vi "Q14070-Z030装调整机构.vi"() -> ()   [LabVIEW 2013]
panel:
  out "error out 4":errorcluster
  out "人工判断不合格状态":bool
  out "涂脂报警状态":string
  out "涂脂报警工步号":dbl
  out "error out 3":errorcluster
  out "型号数量":i32=10
  out "KSJJ":string
  out "FGCS":string
  out "03RFID":string
  out "RFID读取完成":bool
  out "RFID读取触发":bool
  out "芯片ID":string
  out "产品ID":string
  in  "锁紧螺母批次号":string
  in  "调整螺塞批次号":string
  in  "弹簧批次号":string
  in  "O型圈批次号":string
  in  "支撑座批次号":string
  in  "复位按钮":bool
  in  "停止":bool
  in  "联线按钮":bool
  out "通讯状态":bool
  in  "选项卡控件 2":enum32{"自动", "手动", "参数查询"}(tab)
  in  "人工判断\n不合格":bool
  out "本序已做":bool
  out "本序合格":bool
  out "上序不合格":bool
  out "上序合格":bool
  out "取料操作状态":string
  out "取料工步号":dbl
  out "涂脂操作状态":string
  out "涂脂工步号":dbl
  out "流水线操作状态":string
  in  "流水线工步号":dbl
  out "报警提示":string
  out "报警工步号":dbl
  out "I上工位在位":bool
  out "I本工位在位":bool
  out "I下工位在位":bool
  out "I旋转气缸原位  2":bool
  out "I顶升气缸下位 2":bool
  out "I顶升气缸上位  2":bool
  out "I旋转气缸进位 2":bool
  out "I胶瓶在位":bool
  out "I辅具在位":bool
  out "I横孔涂脂在位":bool
  in  "M支撑座手动涂脂有效":bool
  in  "M图像识别涂脂开":bool
  in  "M图像识别触发":bool
  in  "M本工位放行":bool
  in  "M流水线旋转气缸原位":bool
  in  "M上工位放行":bool
  in  "M流水线顶升气缸下降":bool
  in  "M流水线旋转气缸旋转":bool
  in  "M横孔涂脂开":bool
  in  "M流水线顶升气缸顶升":bool
  out "下工位在位":bool
  out "上工位在位":bool
  out "本工位在位":bool
  out "旋转气缸进位":bool
  out "顶升气缸上位":bool
  out "顶升气缸下位":bool
  out "旋转气缸原位":bool
  in  "操作步骤":T1
  in  "参数修改":bool
  in  "参数查询":bool
  in  "参数列表":string[][](table)
  out "员工ID":string
  out "员工姓名":string
  in  "型号选择":u16(ring)=1 items=["J706", "J709", "J728", "J728A", "J728B", "J506X"]
  in  "参数加载":bool
  out "Q场景切换启动2":bool
  out "Q场景切换启动1":bool
  out "备用取料":i16=4
  out "error out 2":errorcluster
  out "ADODB._Connection Out":refnum<k7>
  out "error out":errorcluster
  out "Q场景切换 4":bool
  out "Q场景切换 3":bool
  out "Q场景切换 2":bool
  out "Q场景切换":bool
  out "场景切换选择":i16=4
  out "横孔涂脂设定次数":i16=4
  out "齿条支撑座涂脂设定次数":i16=4
  in  "M备用取料":bool
  out "产品选型":dbl
  # "芜湖机械转向器装配线"
  # "Z030 装调整机构"
  # "Q14070机械转向器装配线"
  # "湖北唯思凌科装备制造有限公司 设计开发 (C)2015"
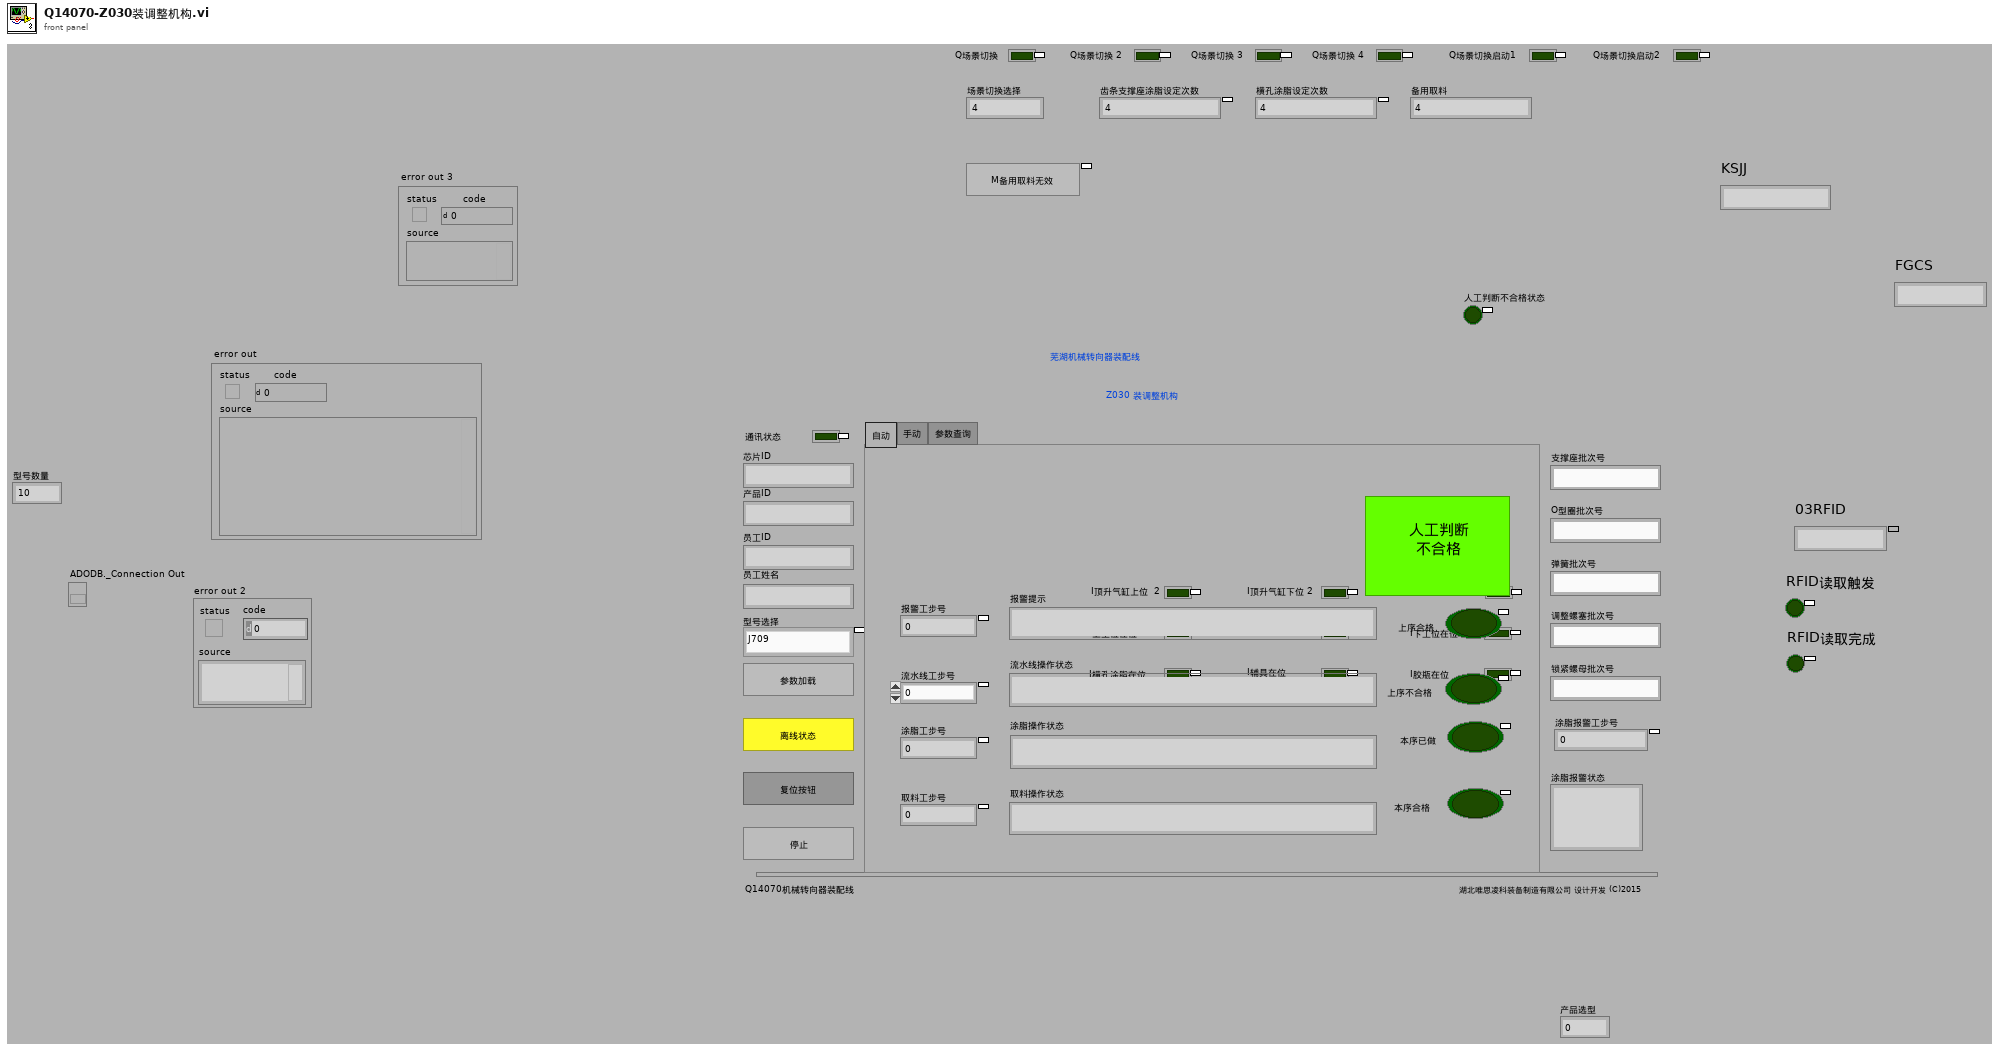
[diagram p1: front panel]
types:
  T1 = cluster{"布尔":bool, "布尔 2":bool, "布尔 3":bool, "布尔 4":bool, "布尔 5":bool, "布尔 6":bool, "布尔 7":bool, "布尔 8":bool}
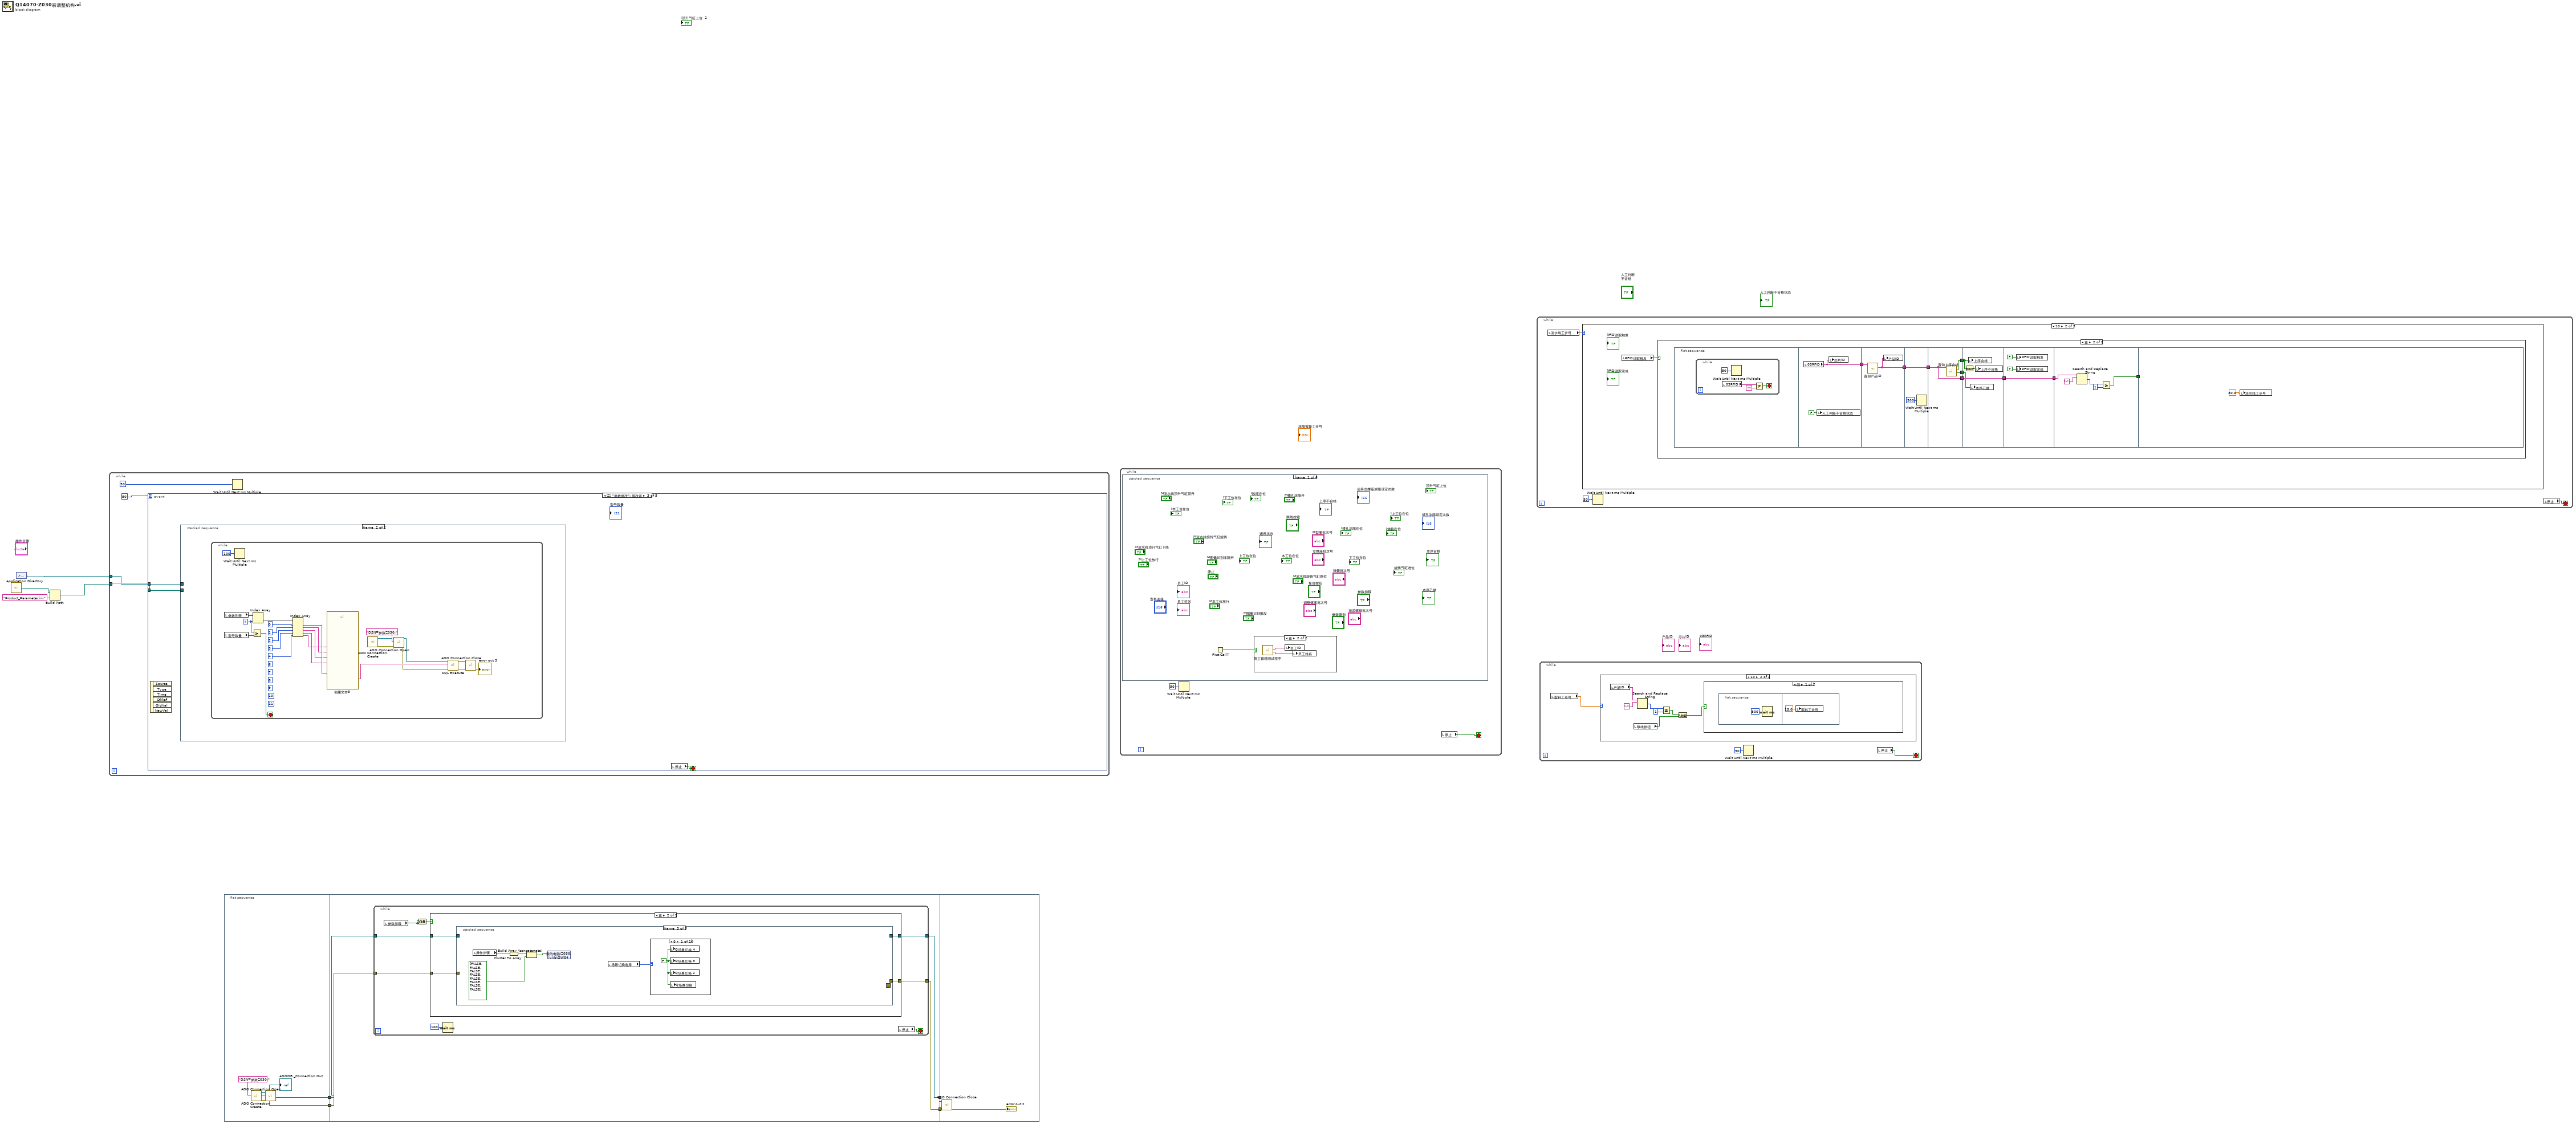
[diagram p0: block diagram]
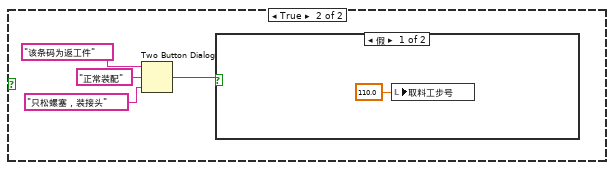
[diagram p3: hidden frame]
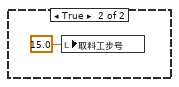
[diagram p4: hidden frame]
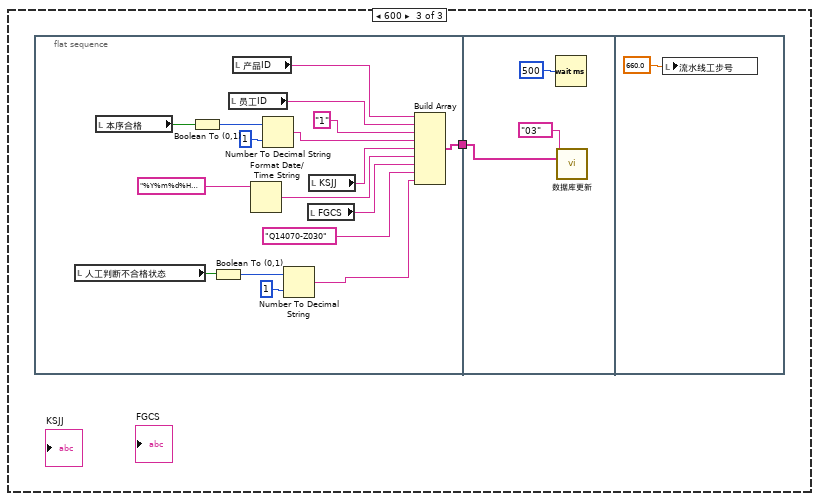
[diagram p7: hidden frame]
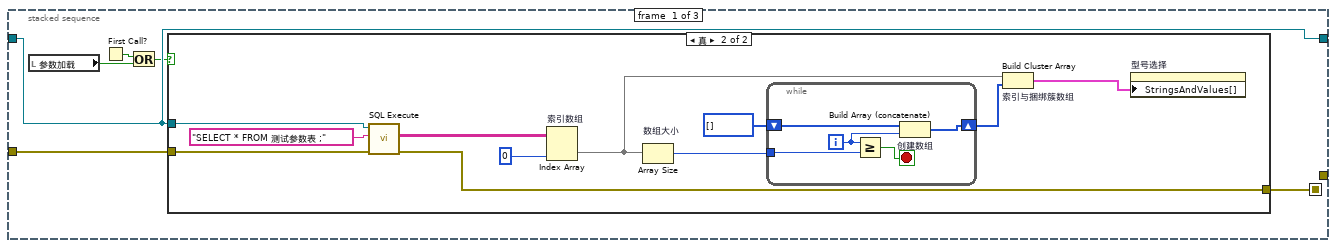
[diagram p9: hidden frame]
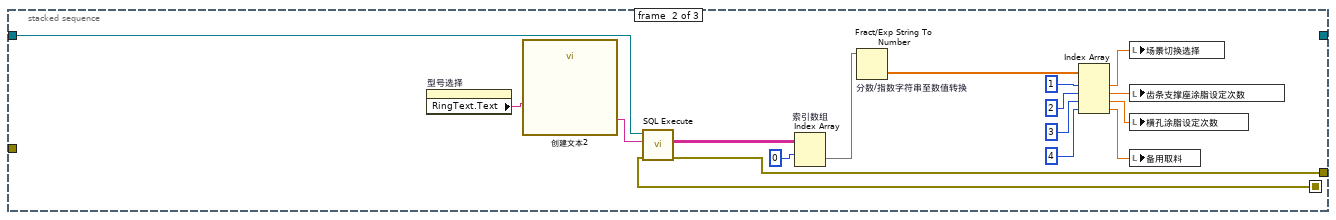
[diagram p11: hidden frame]
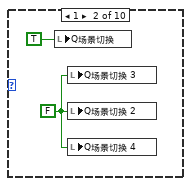
[diagram p12: hidden frame]
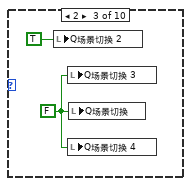
[diagram p13: hidden frame]
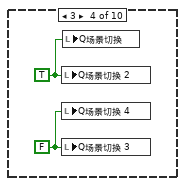
[diagram p14: hidden frame]
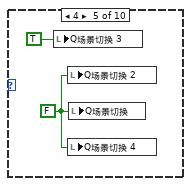
[diagram p15: hidden frame]
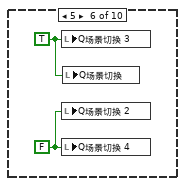
[diagram p16: hidden frame]
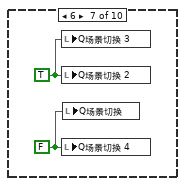
[diagram p17: hidden frame]
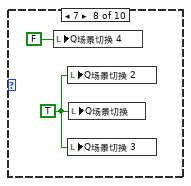
[diagram p18: hidden frame]
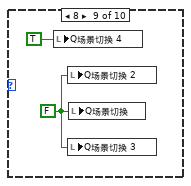
[diagram p19: hidden frame]
diagram:
  n1 = call <vilib>:"Application Directory.vi"() -> ("Application Directory"=w4:path)
  n2 = control-ref of="操作步骤"() -> (w1:refnum<vi>)
  n3 = Build Path(base path=w4, name or relative path="Product_Parameter.ini" ("名称或相对路径")) -> (appended path=w2:path)
  n4 = while {
    tunnel: w1 -> [w12]
    tunnel: w2 -> [w11]
    stop <- w13 stop-if-true
    n5 = event shown="[2] \"参数修改\": 值改变" {
      selector: _ -> [_ _ _ _ _]
      dyn-events: _ -> [_ _ _ _ _]
      timeout: 50 -> [_ _ _ _ _]
      tunnel: w12 -> [_ w28 w62 w95 _]
      tunnel: w11 -> [_ w27 w61 w94 _]
      event Timeout {
        (unwired) 0 ("索引 (行)")
        n6 = event-data() -> ()  [unwired: 3 out]
        n7 = call "ADO Connection Create.vi"() -> ("error out"=w24:errorcluster, "ADODB._Connection Out"=w14:refnum<k7>)  [unwired: 10 in]
        n8 = call "创建文本4"() -> ("Result"=w26:string)  [unwired: 14 in, 1 out]
        n9 = call "ADO Connection Open.vi"("error in (no error)"=w24, "ConnectionString"="DSN=参数Z030;", "ADODB._Connection In"=w14) -> ("error out"=w23:errorcluster, "ADODB._Connection Out"=w15:refnum<k7>)  [unwired: 7 in]
        n10 = call "SQL Execute.vi"("error in (no error)"=w23, "Command Text"=w26, "ADODB._Connection In"=w15) -> ("error out"=w20:errorcluster, "Data"=w22:string[][], "ADODB._Connection Out"=w19:refnum<k7>)  [unwired: 5 in, 1 out]
        n11 = Transpose 2D Array ("二维数组转置")(2D array=w22) -> (transposed array=w21:string[][])
        n12 = Index Array(array=w21) -> (element=w16:string[])  [unwired: 2 in]
        n13 = Array Size(array=w16) -> ()  [unwired: 1 out]
        n14 = control-ref of="型号选择"() -> (w17:refnum<vi>)
        n15 = call "ADO Connection Close.vi"("error in (no error)"=w20, "ADODB._Connection In"=w19) -> ("error out"=→"error out 4":errorcluster)  [unwired: 8 in, 1 out]
        n16 = property class="Ring (严格)"(reference=w17, "Strings []"=w16) -> ()  [unwired: 1 in, 2 out]
      }
      event "参数查询": Value Change {
        n17 = event-data() -> ()  [unwired: 7 out]
        n18 = stacked-sequence {
          tunnel: w28 -> [_ w60]
          tunnel: w27 -> [_ w59]
          frame #0 {
            n19 = flat-sequence {
              tunnel: [w43] -> w34
              tunnel: [w48] -> w33
              tunnel: [w47] -> w32
              tunnel: [w46] -> w31
              tunnel: w34 -> [w53]
              tunnel: w33 -> [w51]
              tunnel: [w52] -> w30
              tunnel: w32 -> [w52]
              tunnel: [w51] -> w29
              tunnel: w31 -> [w50]
              tunnel: w30 -> [w56]
              tunnel: w29 -> [w55]
              frame #0 {
                n20 = call "字符串转换为数组.vi"("查询内容"=",产品型号,场景切换,图像识别位涂脂设定值,横孔涂脂设定值,备用取料有料") -> ("列首"=w35:string[])  [unwired: 10 in]
                n21 = property on="参数列表" class="Tbl (严格)"("Row Headers[]"=w35) -> ()  [unwired: 2 in, 2 out]
              }
              frame #1 {
                n22 = property on="型号选择" class="Ring (严格)"() -> ("RingText.Text"=w42:string)  [unwired: 2 in, 2 out]
                n23 = call "ADO Connection Create.vi"() -> ("error out"=w40:errorcluster, "ADODB._Connection Out"=w39:refnum<k7>)  [unwired: 10 in]
                n24 = call "ADO Connection Open.vi"("error in (no error)"=w40, "ConnectionString"="DSN=参数Z030;", "ADODB._Connection In"=w39) -> ("error out"=w37:errorcluster, "ADODB._Connection Out"=w38:refnum<k7>)  [unwired: 7 in]
                n25 = call "创建文本"("产品型号"=w42) -> ("Result"=w49:string)  [unwired: 13 in, 1 out]
                n26 = call "SQL Execute.vi"("error in (no error)"=w37, "Command Text"=w49, "ADODB._Connection In"=w38) -> ("error out"=w48:errorcluster, "Data"=w45:string[][], "ADODB._Connection Out"=w47:refnum<k7>)  [unwired: 5 in, 1 out]
                n27 = Transpose 2D Array "二维数组转置"(2D array=w45) -> (transposed array=w43:string[][])
                n28 = Index Array(array=w43, index (row)=0 ("索引 (行)")) -> (element=w46:string[])  [unwired: 1 in]
              }
              frame #2 {
                n29 = local write "参数列表"(w53) -> ()
                n30 = property on="参数列表" class="Tbl (严格)"("Column Headers[]"=w50) -> ()  [unwired: 2 in, 2 out]
              }
              frame #3 {
                n31 = call "ADO Connection Close.vi"("error in (no error)"=w55, "ADODB._Connection In"=w56) -> ("error out"=→"error out":errorcluster)  [unwired: 8 in, 1 out]
              }
            }
          }
          frame #1 {
            n32 = property on="型号选择" class="Ring (严格)"() -> ("RingText.Text"=w57:string)  [unwired: 2 in, 2 out]
            n33 = call "Read_Write ParaINI File.vi"("Mode"=enum16{"Read", "Write"}."Read", "Section"=w57, "Filepath"=w59, "Ctl Refnum"=w60) -> ()  [unwired: 7 in, 1 out]
          }
        }
      }
      event "参数修改": Value Change {
        n34 = event-data() -> ()  [unwired: 7 out]
        n35 = stacked-sequence {
          tunnel: w62 -> [w66 _]
          tunnel: w61 -> [w65 _]
          frame #0 {
            n36 = property on="型号选择" class="Ring (严格)"() -> ("RingText.Text"=w64:string)  [unwired: 2 in, 2 out]
            n37 = call "Read_Write ParaINI File.vi"("Mode"=enum16{"Read", "Write"}."Write", "Section"=w64, "Filepath"=w65, "Ctl Refnum"=w66) -> ()  [unwired: 7 in, 1 out]
          }
          frame #1 {
            n38 = while {
              i -> [w88]
              stop <- w87 stop-if-true
              (unwired) 11 ("索引")
              (unwired) 10 ("索引")
              (unwired) 9 ("索引")
              (unwired) 8 ("索引")
              (unwired) 7 ("索引")
              (unwired) 6 ("索引")
              n39 = local read "参数列表"() -> (w90:string[][])
              n40 = local read "型号数量"() -> (w89:i32)
              n41 = Wait Until Next ms Multiple(millisecond multiple=u32 100 ("毫秒倍数")) -> ()  [unwired: 1 out]
              n42 = Greater Or Equal?(x=w88, y=w89) -> (x >= y?=w87:bool)
              n43 = Index Array(array=w90, index (col)=w88) -> (element=w82:string[])  [unwired: 1 in]
              n44 = Index Array(array=w82, index #1=0 ("索引"), index #2=1 ("索引"), index #3=2 ("索引"), index #4=3 ("索引"), index #5=4 ("索引")) -> (element #1=w77:string, element #2=w76:string, element #3=w75:string, element #4=w74:string, element #5=w73:string)
              n45 = call "创建文本3"("备用取料有料"=w73, "场景切换"=w76, "图像识别位涂脂设定值"=w75, "横孔涂脂设定值"=w74, "产品型号"=w77) -> ("Result"=w79:string)  [unwired: 9 in, 1 out]
              n46 = call "ADO Connection Create.vi"() -> ("error out"=w70:errorcluster, "ADODB._Connection Out"=w69:refnum<k7>)  [unwired: 10 in]
              n47 = call "ADO Connection Open.vi"("error in (no error)"=w70, "ConnectionString"="DSN=参数Z030;", "ADODB._Connection In"=w69) -> ("error out"=w67:errorcluster, "ADODB._Connection Out"=w68:refnum<k7>)  [unwired: 7 in]
              n48 = call "SQL Execute.vi"("error in (no error)"=w67, "Command Text"=w79, "ADODB._Connection In"=w68) -> ("error out"=w80:errorcluster, "ADODB._Connection Out"=w81:refnum<k7>)  [unwired: 5 in, 2 out]
              n49 = call "ADO Connection Close.vi"("error in (no error)"=w80, "ADODB._Connection In"=w81) -> ("error out"=→"error out 3":errorcluster)  [unwired: 8 in, 1 out]
            }
          }
        }
      }
      event "型号选择": Value Change {
        n50 = event-data() -> ()  [unwired: 7 out]
        n51 = property on="型号选择" class="Ring (严格)"() -> ("RingText.Text"=w92:string)  [unwired: 2 in, 2 out]
        n52 = call "Read_Write ParaINI File.vi"("Mode"=enum16{"Read", "Write"}."Read", "Section"=w92, "Filepath"=w94, "Ctl Refnum"=w95) -> ()  [unwired: 7 in, 1 out]
      }
      event "停止": Value Change {
        n53 = event-data() -> ()  [unwired: 7 out]
        n54 = flat-sequence {
          frame #0 {
            n55 = local write "涂脂工步号"(0.0 ("工步号")) -> ()
          }
          frame #1 {
            n56 = Wait Until Next ms Multiple(millisecond multiple=u32 1000 ("毫秒倍数")) -> ()  [unwired: 1 out]
          }
          frame #2 {
            n57 = Quit LabVIEW(quit? (T)=TRUE ("停止？(T)")) -> ()
          }
        }
      }
    }
    n58 = Wait Until Next ms Multiple(millisecond multiple=u32 50 ("毫秒倍数")) -> ()  [unwired: 1 out]
    n59 = local read "停止"() -> (w13:bool)
  }
  n60 = flat-sequence {
    tunnel: [w100] -> w8
    tunnel: [w99] -> w7
    tunnel: w8 -> [w107]
    tunnel: w7 -> [w106]
    tunnel: [w105] -> w6
    tunnel: [w104] -> w5
    tunnel: w6 -> [w185]
    tunnel: w5 -> [w184]
    frame #0 {
      n61 = call "ADO Connection Create.vi"() -> ("error out"=w102:errorcluster, "ADODB._Connection Out"=w103:refnum<k7>)  [unwired: 10 in]
      n62 = call "ADO Connection Open.vi"("error in (no error)"=w102, "ConnectionString"="DSN=参数Z030;", "ADODB._Connection In"=w103) -> ("error out"=w99:errorcluster, "ADODB._Connection Out"=w100:refnum<k7>)  [unwired: 7 in]
      "ADODB._Connection Out" <- w100
    }
    frame #1 {
      n63 = while {
        tunnel: w107 -> [w112]
        tunnel: w106 -> [w111]
        tunnel: [w110] -> w105
        tunnel: [w109] -> w104
        stop <- w114 stop-if-true
        n64 = local read "参数加载"() -> (w108:bool)
        n65 = Or(x=w108, y=w108) -> (x .or. y?=w113:bool)
        n66 = case shown="真" w113 {
          tunnel: w112 -> [w117 w121]
          tunnel: w111 -> [w116 w120]
          tunnel: [w117 w119] -> w110
          tunnel: [w116 w118] -> w109
          frame False {
          }
          frame True {
            n67 = stacked-sequence {
              seq-local: [w125 _ _] -> [_ w159 _]
              tunnel: w121 -> [w126 w156 _]
              tunnel: w120 -> [w127 _ _]
              tunnel: [w126 _ _] -> w119
              tunnel: [_ w158 _] -> w118
              frame #0 {
                n68 = local read "参数加载"() -> (w123:bool)
                n69 = First Call?() -> (First Call?: T/F=w124:bool)
                n70 = Or(x=w124, y=w123) -> (x .or. y?=w122:bool)
                n71 = case shown="真" w122 {
                  tunnel: w127 -> [w128 w133]
                  tunnel: w126 -> [_ w131]
                  tunnel: [w128 w130] -> w125
                  frame False {
                  }
                  frame True {
                    n72 = call "SQL Execute.vi"("error in (no error)"=w133, "Command Text"="SELECT * FROM 测试参数表 ;", "ADODB._Connection In"=w131) -> ("error out"=w130:errorcluster, "Data"=w134:string[][])  [unwired: 5 in, 2 out]
                    n73 = Index Array "索引数组"(array=w134, index (col)=0 ("禁用的索引 (列)")) -> (element=w137:string[])  [unwired: 1 in]
                    n74 = Array Size "数组大小"(array=w137) -> (size(s)=w136:i32)
                    n75 = while {
                      shift-right: [w142] -> w135
                      shift-left: i32[] [] -> [w143]
                      tunnel: w136 -> [w140]
                      i -> [w141]
                      stop <- w144 stop-if-true
                      n76 = Greater Or Equal?(x=w141, y=w140) -> (x >= y?=w144:bool)
                      n77 = Build Array (concatenate) "创建数组"(w143, w141) -> (w142:i32[])
                    }
                    n78 = Build Cluster Array "索引与捆绑簇数组"(w137, w135) -> (w129:cluster{"String":string, i32}[])
                    n79 = property on="型号选择" class="Ring (严格)"("StringsAndValues[]"=w129) -> ()  [unwired: 2 in, 2 out]
                  }
                }
              }
              frame #1 {
                n80 = property on="型号选择" class="Ring (严格)"() -> ("RingText.Text"=w155:string)  [unwired: 2 in, 2 out]
                n81 = call "创建文本2"("产品型号"=w155) -> ("Result"=w157:string)  [unwired: 13 in, 1 out]
                n82 = call "SQL Execute.vi"("error in (no error)"=w159, "Command Text"=w157, "ADODB._Connection In"=w156) -> ("error out"=w158:errorcluster, "Data"=w161:string[][])  [unwired: 5 in, 2 out]
                n83 = Index Array "索引数组"(array=w161, index (row)=0 ("索引 (行)")) -> (element=w154:string[])  [unwired: 1 in]
                n84 = Fract/Exp String To Number "分数/指数字符串至数值转换"(string=w154) -> (number=w149:dbl[])  [unwired: 3 in, 1 out]
                n85 = Index Array(array=w149, index #1=1 ("索引"), index #2=2 ("索引"), index #3=3 ("索引"), index #4=4 ("索引")) -> (element #1=w148:dbl, element #2=w147:dbl, element #3=w146:dbl, element #4=w145:dbl)
                n86 = local write "场景切换选择"(w148) -> ()
                n87 = local write "齿条支撑座涂脂设定次数"(w147) -> ()
                n88 = local write "横孔涂脂设定次数"(w146) -> ()
                n89 = local write "备用取料"(w145) -> ()
              }
              frame #2 {
                n90 = local read "操作步骤"() -> (w165:T1)
                n91 = Cluster To Array(cluster=w165) -> (array=w164:bool[])
                n92 = Build Array (concatenate)(w164, bool[] [FALSE, FALSE, FALSE, FALSE, FALSE, FALSE, FALSE, FALSE]) -> (w163:bool[])
                n93 = shared-variable "我的电脑\\Z030.lvlib\\QW04"(w163) -> ()  [unwired: 1 in, 1 out]
                n94 = local read "场景切换选择"() -> (w166:i16)
                n95 = case shown="0" w166 {
                  frame 0 {
                    w167 = FALSE
                    n96 = local write "Q场景切换 4"(w167) -> ()
                    n97 = local write "Q场景切换 3"(w167) -> ()
                    n98 = local write "Q场景切换 2"(w167) -> ()
                    n99 = local write "Q场景切换"(w167) -> ()
                  }
                  frame 1 {
                    w169 = FALSE
                    n100 = local write "Q场景切换"(TRUE ("Q场景切换")) -> ()
                    n101 = local write "Q场景切换 3"(w169) -> ()
                    n102 = local write "Q场景切换 2"(w169) -> ()
                    n103 = local write "Q场景切换 4"(w169) -> ()
                  }
                  frame 2 {
                    w170 = FALSE
                    n104 = local write "Q场景切换 2"(TRUE ("Q场景切换")) -> ()
                    n105 = local write "Q场景切换 3"(w170) -> ()
                    n106 = local write "Q场景切换 4"(w170) -> ()
                    n107 = local write "Q场景切换"(w170) -> ()
                  }
                  frame 3 {
                    w173 = TRUE ("Q场景切换")
                    w172 = FALSE
                    n108 = local write "Q场景切换 2"(w173) -> ()
                    n109 = local write "Q场景切换 4"(w172) -> ()
                    n110 = local write "Q场景切换 3"(w172) -> ()
                    n111 = local write "Q场景切换"(w173) -> ()
                  }
                  frame 4 {
                    w174 = FALSE
                    n112 = local write "Q场景切换 3"(TRUE ("Q场景切换")) -> ()
                    n113 = local write "Q场景切换 2"(w174) -> ()
                    n114 = local write "Q场景切换 4"(w174) -> ()
                    n115 = local write "Q场景切换"(w174) -> ()
                  }
                  frame 5 {
                    w177 = TRUE ("Q场景切换")
                    w176 = FALSE
                    n116 = local write "Q场景切换 3"(w177) -> ()
                    n117 = local write "Q场景切换 2"(w176) -> ()
                    n118 = local write "Q场景切换 4"(w176) -> ()
                    n119 = local write "Q场景切换"(w177) -> ()
                  }
                  frame 6 {
                    w179 = TRUE ("Q场景切换")
                    w178 = FALSE
                    n120 = local write "Q场景切换 3"(w179) -> ()
                    n121 = local write "Q场景切换 2"(w179) -> ()
                    n122 = local write "Q场景切换 4"(w178) -> ()
                    n123 = local write "Q场景切换"(w178) -> ()
                  }
                  frame 7 {
                    w181 = TRUE ("Q场景切换")
                    n124 = local write "Q场景切换 4"(FALSE) -> ()
                    n125 = local write "Q场景切换 2"(w181) -> ()
                    n126 = local write "Q场景切换 3"(w181) -> ()
                    n127 = local write "Q场景切换"(w181) -> ()
                  }
                  frame 8 {
                    w182 = FALSE
                    n128 = local write "Q场景切换 4"(TRUE ("Q场景切换")) -> ()
                    n129 = local write "Q场景切换 2"(w182) -> ()
                    n130 = local write "Q场景切换 3"(w182) -> ()
                    n131 = local write "Q场景切换"(w182) -> ()
                  }
                  frame 32, Default {
                  }
                }
              }
            }
          }
        }
        n132 = Wait (ms)(milliseconds to wait=u32 100 ("等待时间（毫秒）")) -> ()  [unwired: 1 out]
        n133 = local read "停止"() -> (w114:bool)
      }
    }
    frame #2 {
      n134 = call "ADO Connection Close.vi"("error in (no error)"=w184, "ADODB._Connection In"=w185) -> ("error out"=→"error out 2":errorcluster)  [unwired: 8 in, 1 out]
    }
  }
  n135 = while {
    stop <- w187 stop-if-true
    n136 = stacked-sequence {
      frame #0 {
        n137 = First Call?() -> (First Call?: T/F=w189:bool)
        n138 = case shown="真" w189 {
          frame False {
          }
          frame True {
            n139 = call "员工管理测试程序.vi"() -> ("员工姓名"=w191:string, "员工ID"=w190:string)  [unwired: 10 in]
            n140 = local write "员工ID"(w190) -> ()
            n141 = local write "员工姓名"(w191) -> ()
          }
        }
      }
      frame #1 {
      }
      frame #2 {
        n142 = local read "流水线工步号"() -> (w199:dbl)
        n143 = local read "取料工步号"() -> (w195:dbl)
        n144 = local read "涂脂工步号"() -> (w196:dbl)
        n145 = local read "报警工步号"() -> (w193:dbl)
        n146 = case shown="90" w195 {
          tunnel: ["等待流水线准备好" ("工步操作状态") "取辅具放到横孔" ("工步操作状态") "取涂脂头放到横孔" ("工步操作状态") "按横孔涂脂按钮" ("工步操作状态") "涂脂头归位，辅具归位" ("工步操作状态") "  等待支撑座涂脂完成信号" ("工步操作状态") " 取调整螺塞" ("工步操作状态") " 取调整螺塞胶" ("工步操作状态") "放回调整螺塞胶" ("工步操作状态") "80 取弹簧" ("工步操作状态") "" ("工步操作状态") "气动扳手拧紧" ("工步操作状态") "100 取锁紧螺母" ("工步操作状态") " 定扭扳手定扭" ("工步操作状态") "120 取料完成" ("工步操作状态") "循环结束" ("工步操作状态")] -> w194
          frame 0, Default {
          }
          frame 10 {
          }
          frame 20 {
          }
          frame 30 {
          }
          frame 40 {
          }
          frame 50 {
          }
          frame 70 {
          }
          frame 75 {
          }
          frame 77 {
          }
          frame 80 {
          }
          frame 85 {
          }
          frame 90 {
          }
          frame 100 {
          }
          frame 110 {
          }
          frame 120 {
          }
          frame 990 {
          }
        }
        "取料操作状态" <- w194
        n147 = case shown="990" w196 {
          tunnel: ["等待涂脂启动" ("工步操作状态") "10 取齿条支撑座总成" ("工步操作状态") "20 取O型圈" ("工步操作状态") "25 按涂脂按钮" ("工步操作状态") "30 检测工件有无" ("工步操作状态") " 手动下按支撑座涂脂按钮" ("工步操作状态") "40  自动涂脂" ("工步操作状态") "循环结束" ("工步操作状态")] -> w197
          frame 0, Default {
          }
          frame 10 {
          }
          frame 20 {
          }
          frame 25 {
          }
          frame 30 {
          }
          frame 35 {
          }
          frame 40 {
          }
          frame 990 {
          }
        }
        "涂脂操作状态" <- w197
        n148 = case shown="800" w199 {
          tunnel: ["等待启动" ("工步操作状态") "RFID读取触发" ("工步操作状态") "" ("工步操作状态") "上序合格判断" ("工步操作状态") "" ("工步操作状态") "上阻挡器放行" ("工步操作状态") "本工位在位检测" ("工步操作状态") "流水线顶升" ("工步操作状态") "流水线夹具旋转" ("工步操作状态") "流水线准备好,等待取料完成信号" ("工步操作状态") "等待取料完成" ("工步操作状态") "给出本工位合格和完成信号" ("工步操作状态") "按下放行按钮后，夹具旋转" ("工步操作状态") "流水线顶升气缸下降" ("工步操作状态") "本工位放行" ("工步操作状态") "本工位放行完成" ("工步操作状态") "数据上传完成" ("工步操作状态") "本序已做，请复位" ("工步操作状态") "循环结束" ("工步操作状态")] -> w198
          frame 0, Default {
          }
          frame 10 {
          }
          frame 20 {
          }
          frame 30 {
          }
          frame 40 {
          }
          frame 70 {
          }
          frame 80 {
          }
          frame 95 {
          }
          frame 100 {
          }
          frame 200 {
          }
          frame 500 {
          }
          frame 520 {
          }
          frame 540 {
          }
          frame 550 {
          }
          frame 560 {
          }
          frame 580 {
          }
          frame 660 {
          }
          frame 800 {
          }
          frame 990 {
          }
        }
        "流水线操作状态" <- w198
        n149 = case shown="1" w193 {
          tunnel: ["无报警信息" ("工步操作状态") "急停被按下" ("工步操作状态") "取辅具放到横孔" ("工步操作状态") "取涂脂头放到横孔" ("工步操作状态") "按启动按钮" ("工步操作状态") "涂脂头归位，辅具归位" ("工步操作状态") "50  等待涂脂工位2完成信号" ("工步操作状态") " 取弹簧" ("工步操作状态") "80 取调整螺塞" ("工步操作状态") "90 气动扳手拧紧" ("工步操作状态") "100 取锁紧螺母" ("工步操作状态") "110 定扭扳手定扭" ("工步操作状态") "120 取料完成" ("工步操作状态") "循环结束" ("工步操作状态")] -> w192
          frame 0, Default {
          }
          frame 1 {
          }
          frame 10 {
          }
          frame 20 {
          }
          frame 30 {
          }
          frame 40 {
          }
          frame 50 {
          }
          frame 70 {
          }
          frame 80 {
          }
          frame 90 {
          }
          frame 100 {
          }
          frame 110 {
          }
          frame 120 {
          }
          frame 990 {
          }
        }
        "报警提示" <- w192
      }
      frame #3 {
        n150 = local read "涂脂报警工步号"() -> (w258:dbl)
        n151 = case shown="0, 默认" w258 {
          tunnel: ["工作正常" "横孔涂脂报警，请加脂" "支撑座涂脂报警，请加脂"] -> w257
          frame 0, Default {
          }
          frame 11 {
          }
          frame 12 {
          }
        }
        "涂脂报警状态" <- w257
      }
      frame #4 {
        n152 = disable-structure shown="禁用" {
          frame Disabled {
            n153 = local read "备用取料"() -> (w269:i16)
            n154 = case shown="0" w269 {
              frame 0 {
                n155 = local write "M备用取料"(FALSE ("M备用取料")) -> ()
              }
              frame 1 {
                n156 = local write "M备用取料"(TRUE ("M备用取料")) -> ()
              }
              frame 2, Default {
              }
            }
          }
          frame Enabled {
          }
        }
        n157 = local read "人工判断\n不合格"() -> (w266:bool)
        n158 = local read "取料工步号"() -> (w265:dbl)
        n159 = Greater Or Equal?(x=w265, y=70.0) -> (x >= y?=w267:bool)
        n160 = Less Or Equal?(x=w265, y=110.0) -> (x <= y?=w263:bool)
        n161 = Compound Arithmetic op=AND(w267, w263, w266) -> (w262:bool)
        n162 = case shown="真" w262 {
          frame False {
          }
          frame True {
            n163 = local write "人工判断不合格状态"(TRUE ("人工判断不合格状态")) -> ()
          }
        }
      }
      frame #5 {
        n164 = local read "参数加载"() -> (w273:bool)
        n165 = case shown="真" w273 {
          frame False {
          }
          frame True {
            n166 = flat-sequence {
              frame #0 {
                n167 = Wait Until Next ms Multiple(millisecond multiple=u32 1000 ("毫秒计时值")) -> ()  [unwired: 1 out]
              }
              frame #1 {
                w275 = TRUE
                "Q场景切换启动2" <- w275
                "Q场景切换启动1" <- w275
              }
              frame #2 {
                n168 = Wait Until Next ms Multiple(millisecond multiple=u32 1000 ("毫秒计时值")) -> ()  [unwired: 1 out]
              }
              frame #3 {
                w277 = FALSE
                n169 = local write "Q场景切换启动1"(w277) -> ()
                n170 = local write "Q场景切换启动2"(w277) -> ()
              }
            }
          }
        }
      }
    }
    n171 = Wait Until Next ms Multiple(millisecond multiple=u32 50 ("毫秒倍数")) -> ()  [unwired: 1 out]
    n172 = local read "停止"() -> (w187:bool)
  }
  n173 = while {
    stop <- w279 stop-if-true
    n174 = local read "流水线工步号"() -> (w278:dbl)
    n175 = case shown="10" w278 {
      frame 0, Default {
      }
      frame 10 {
        n176 = local read "RFID读取触发"() -> (w281:bool)
        n177 = case shown="真" w281 {
          frame False {
          }
          frame True {
            n178 = flat-sequence {
              tunnel: [w296] -> w290
              tunnel: w290 -> [w298]
              tunnel: [w297] -> w283
              tunnel: w283 -> [w300]
              tunnel: [w300] -> w282
              tunnel: w282 -> [w301]
              tunnel: [w303] -> w289
              tunnel: [w302] -> w288
              tunnel: [w301] -> w287
              tunnel: w289 -> [w305]
              tunnel: w288 -> [w304]
              tunnel: w287 -> [w307]
              tunnel: [w307] -> w286
              tunnel: w286 -> [w308]
              tunnel: [w308] -> w285
              tunnel: w285 -> [w315]
              tunnel: [w311] -> w284
              tunnel: w284 -> [_]
              frame #0 {
                n179 = while {
                  stop <- w292 stop-if-true
                  n180 = local read "03RFID"() -> (w294:string)
                  n181 = Wait Until Next ms Multiple(millisecond multiple=u32 50 ("毫秒倍数")) -> ()  [unwired: 1 out]
                  n182 = Not Equal?(x=w294, y="") -> (x != y?=w292:bool)
                }
              }
              frame #1 {
                n183 = local read "03RFID"() -> (w296:string)
                n184 = local write "人工判断不合格状态"(FALSE ("人工判断不合格状态")) -> ()
                n185 = local write "芯片ID"(w296) -> ()
              }
              frame #2 {
                n186 = call "查询产品ID.vi"("芯片编码"=w298) -> ("产品ID"=w297:string)  [unwired: 8 in, 2 out]
                n187 = local write "产品ID"(w297) -> ()
              }
              frame #3 {
                n188 = Wait Until Next ms Multiple(millisecond multiple=u32 500 ("毫秒倍数")) -> ()  [unwired: 1 out]
              }
              frame #4 {
                n189 = call "查询上序合格.vi"("产品ID"=w301) -> ("本序已做"=w302:bool, "上序合格"=w303:bool)  [unwired: 8 in, 1 out]
              }
              frame #5 {
                n190 = Not(x=w305) -> (.not. x?=w306:bool)
                n191 = local write "上序合格"(w305) -> ()
                n192 = local write "本序已做"(w304) -> ()
                n193 = local write "上序不合格"(w306) -> ()
              }
              frame #6 {
                n194 = local write "RFID读取触发"(FALSE ("RFID读取触发")) -> ()
                n195 = local write "RFID读取完成"(TRUE ("RFID读取完成")) -> ()
              }
              frame #7 {
                n196 = Search and Replace String(input string=w315, search string="-" ("搜索字符串")) -> (number of replacements=w313:i32)  [unwired: 6 in, 3 out]
                n197 = Greater Or Equal?(x=w313, y=1) -> (x >= y?=w311:bool)
              }
              frame #8 {
                n198 = local write "流水线工步号"(30.0 ("工步号")) -> ()
              }
            }
          }
        }
      }
      frame 600 {
        n199 = flat-sequence {
          tunnel: [w325] -> w317
          tunnel: w317 -> [w335]
          frame #0 {
            n200 = local read "人工判断不合格状态"() -> (w319:bool)
            n201 = local read "本序合格"() -> (w330:bool)
            n202 = Boolean To (0,1)(Boolean=w330) -> (0, 1=w334:i16)
            n203 = Boolean To (0,1)(Boolean=w319) -> (0, 1=w320:i16)
            n204 = local read "员工ID"() -> (w331:string)
            n205 = local read "产品ID"() -> (w324:string)
            n206 = Format Date/Time String(time format string (%c)="%Y%m%d%H%M" ("时间格式字符串(%c)")) -> (date/time string=w332:string)  [unwired: 2 in]
            n207 = Number To Decimal String(number=w334, width (-)=i16 1 ("宽度(-)")) -> (decimal integer string=w322:string)
            n208 = Number To Decimal String(number=w320, width (-)=i16 1 ("宽度(-)")) -> (decimal integer string=w318:string)
            n209 = local read "FGCS"() -> (w327:string)
            n210 = local read "KSJJ"() -> (w329:string)
            n211 = Build Array(w324, w331, "1" ("元素"), w322, w329, w332, w327, "Q14070-Z030", w318) -> (w325:string[])
          }
          frame #1 {
            n212 = Wait (ms)(milliseconds to wait=u32 500 ("等待时间（毫秒）")) -> ()  [unwired: 1 out]
            n213 = call "数据库更新.vi"("设备号"="03", "数据"=w335) -> ()  [unwired: 13 in, 1 out]
          }
          frame #2 {
            n214 = local write "流水线工步号"(660.0 ("工步号")) -> ()
          }
        }
      }
    }
    n215 = Wait Until Next ms Multiple(millisecond multiple=u32 50 ("毫秒倍数")) -> ()  [unwired: 1 out]
    n216 = local read "停止"() -> (w279:bool)
  }
  n217 = while {
    stop <- w340 stop-if-true
    n218 = local read "取料工步号"() -> (w339:dbl)
    n219 = case shown="10" w339 {
      frame 0, Default {
      }
      frame 10 {
        n220 = local read "产品ID"() -> (w345:string)
        n221 = local read "联线按钮"() -> (w343:bool)
        n222 = Search and Replace String(input string=w345, search string="-" ("搜索字符串")) -> (number of replacements=w347:i32)  [unwired: 6 in, 3 out]
        n223 = Greater Or Equal?(x=w347, y=1) -> (x >= y?=w344:bool)
        n224 = And(x=w344, y=w343) -> (x .and. y?=w342:bool)
        n225 = case shown="假" w342 {
          frame False {
            n226 = flat-sequence {
              frame #0 {
                n227 = Wait (ms)(milliseconds to wait=u32 500 ("等待时间（毫秒）")) -> ()  [unwired: 1 out]
              }
              frame #1 {
                n228 = local write "取料工步号"(15.0 ("取料工步号")) -> ()
              }
            }
          }
          frame True {
            n229 = Two Button Dialog(message="该条码为返工件" ("消息"), 1:"只松螺塞，装接头" ("F按钮名称（“取消”）"), 2:"正常装配" ("T按钮名称（“确定”）")) -> (T button?=w351:bool)
            n230 = case shown="假" w351 {
              frame False {
                n231 = local write "取料工步号"(110.0 ("取料工步号")) -> ()
              }
              frame True {
                n232 = local write "取料工步号"(15.0 ("取料工步号")) -> ()
              }
            }
          }
        }
      }
    }
    n233 = Wait Until Next ms Multiple(millisecond multiple=u32 50 ("毫秒倍数")) -> ()  [unwired: 1 out]
    n234 = local read "停止"() -> (w340:bool)
  }
